vi "SV RMS Average Spectra (Real).vi"(0 "real spectra":cluster{"f0":dbl, "df":dbl, "magnitude":dbl[]}[](array[cluster]) {"magnitude" format="%.2p"; "df" format="%.2p"; "f0" format="%.2p"}, 4 "spectrum info":T1={"channel name"="", "description"="", "x-axis units"=0, "spectral info"={"spectrum type"=enum."Power [Magnitude^2]", "linear/dB"=enum."linear", "window"=0, "window size"=0, "FFT size"=0}, "engineering units"=1, "custom label"="", "dB reference [EU]"=0.0, "peak units"=enum."rms", "weighting filter"=0, "spectral density?"=FALSE, "unit label"="", "spectrum skewed?"=FALSE, "complimentary spectrum units"=enum."none"} {"x-axis units" items=["Time (s)"=0, "Frequency-CB (Hz)"=1, "Frequency-CPB (Hz)"=1248, "Frequency-Arbitrary (Hz)"=2357, "Quefrency (s)"=2, "Revolutions (rev)"=3, "Order"=4, "Speed (RPM)"=11, "Speed (rad/s)"=21, "Index"=65535]; "weighting filter" items=["Linear", "A-weighting", "B-weighting", "C-weighting", "ITU-R 468-4", "Dolby", "CCITT", "C-message", "Wb", "Wc", "Wd", "We", "Wf", "Wh", "Wj", "Wk", "Wm", "AES17 20 kHz lowpass", "AES17 40 kHz lowpass", "AES17 20 kHz highpass", "AES17 40 kHz highpass"]; "dB reference [EU]" format="%.2f"; "engineering units" items=["custom..."=0, "V"=1, "A"=21, "C"=30, "pC"=31, "s"=32, "-"=29, "Pa"=2, "N"=20, "g"=3, "m/s^2"=4, "m/s"=5, "m"=6, "mm/s"=12, "mm"=13, "micron/s"=14, "micron"=15, "in/s^2"=7, "in/s"=8, "in"=9, "mil/s"=10, "mil"=11, "rad/s^2"=16, "rad/s"=17, "rad"=18, "deg/s^2"=26, "deg/s"=27, "deg"=28, "RPM"=22, "cycle/s^2"=23, "Hz"=24, "cycle"=25, "strain"=19]; "spectral info"."window" items=["None "=0, "Hanning"=1, "Hamming"=2, "Blackman-Harris"=3, "Exact Blackman"=4, "Blackman"=5, "Flat Top"=6, "4 Term B-Harris "=7, "7 Term B-Harris"=8, "Low Sidelobe"=9, "Force - Exponential"=10, "Gaussian"=62]}, 5 "error in (no error)":errorcluster) -> (13 "averages completed":dbl, 14 "rms average spectrum":cluster{"f0":dbl, "df":dbl, "magnitude":dbl[]} {"magnitude" format="%.2p"; "df" format="%.2p"; "f0" format="%.2p"}, 15 "unit label":string, 18 "spectrum info":T1={"channel name"="", "description"="", "x-axis units"=0, "spectral info"={"spectrum type"=enum."Power [Magnitude^2]", "linear/dB"=enum."linear", "window"=0, "window size"=0, "FFT size"=0}, "engineering units"=1, "custom label"="", "dB reference [EU]"=0.0, "peak units"=enum."rms", "weighting filter"=0, "spectral density?"=FALSE, "unit label"="", "spectrum skewed?"=FALSE, "complimentary spectrum units"=enum."none"} {"x-axis units" items=["Time (s)"=0, "Frequency-CB (Hz)"=1, "Frequency-CPB (Hz)"=1248, "Frequency-Arbitrary (Hz)"=2357, "Quefrency (s)"=2, "Revolutions (rev)"=3, "Order"=4, "Speed (RPM)"=11, "Speed (rad/s)"=21, "Index"=65535]; "weighting filter" items=["Linear", "A-weighting", "B-weighting", "C-weighting", "ITU-R 468-4", "Dolby", "CCITT", "C-message", "Wb", "Wc", "Wd", "We", "Wf", "Wh", "Wj", "Wk", "Wm", "AES17 20 kHz lowpass", "AES17 40 kHz lowpass", "AES17 20 kHz highpass", "AES17 40 kHz highpass"]; "dB reference [EU]" format="%.2f"; "engineering units" items=["custom..."=0, "V"=1, "A"=21, "C"=30, "pC"=31, "s"=32, "-"=29, "Pa"=2, "N"=20, "g"=3, "m/s^2"=4, "m/s"=5, "m"=6, "mm/s"=12, "mm"=13, "micron/s"=14, "micron"=15, "in/s^2"=7, "in/s"=8, "in"=9, "mil/s"=10, "mil"=11, "rad/s^2"=16, "rad/s"=17, "rad"=18, "deg/s^2"=26, "deg/s"=27, "deg"=28, "RPM"=22, "cycle/s^2"=23, "Hz"=24, "cycle"=25, "strain"=19]; "spectral info"."window" items=["None "=0, "Hanning"=1, "Hamming"=2, "Blackman-Harris"=3, "Exact Blackman"=4, "Blackman"=5, "Flat Top"=6, "4 Term B-Harris "=7, "7 Term B-Harris"=8, "Low Sidelobe"=9, "Force - Exponential"=10, "Gaussian"=62]}, 19 "error out":errorcluster)   [LabVIEW 2017]
doc: "Computes the linear RMS-averaged power spectrum of <B>scaled signal [EU]</B> in a linear scale. Use the power spectrum to quantify signal components as a function of frequency. Use this VI on embedded targets that have limited computational resources. Wire data to the <B>scaled signal [EU]</B> input to determine the polymorphic instance to use or manually select the instance."
uses:
  <vilib>/addons/_NISVFA/_Shared subVIs/Controls/svc_Spectrum Info.ctl
  <vilib>/addons/_NISVFA/_Shared subVIs/Controls/svc_X-Axis Units.ctl
  <vilib>/addons/_NISVFA/_Shared subVIs/Controls/svc_Spectrum Type.ctl
  <vilib>/addons/_NISVFA/_Shared subVIs/Controls/svc_Engineering Units Text Ring.ctl
  <vilib>/addons/_NISVFA/_Shared subVIs/Controls/svc_Weighting Filter Text Ring.ctl
  <vilib>/addons/_NISVFA/_Shared subVIs/Controls/svc_Complimentary Spectrum Units.ctl
  <vilib>/addons/_NISVFA/_Spectrum Processing/SVFA Unit Conversion (1 Ch).vi
  <vilib>/addons/_NISVFA/_Shared subVIs/Common/svc_Spectrum Units.vi
  <vilib>/addons/_NISVFA/_Spectrum Processing/subVIs/svfa_Conversion Utility (spectrum info).vi
  <vilib>/addons/_NISVFA/_Spectrum Processing/subVIs/svfa_Peak to RMS to Peak2Peak.vi
  <vilib>/addons/_NISVFA/_Spectrum Processing/subVIs/svfa_Mag to Mag2.vi
  <vilib>/addons/_NISVFA/_Spectrum Processing/subVIs/svfa_Linear to dB.vi
  <vilib>/addons/_NISVFA/_Spectrum Processing/subVIs/svfa_dBrefA to dBrefB.vi
  <vilib>/addons/_NISVFA/_Spectrum Processing/subVIs/svfa_Spectrum to Spectral Density.vi
  <vilib>/addons/_NISVFA/_Shared subVIs/Common/svc_Get Weighting Enum and Labels.vi
  <vilib>/addons/_NISVFA/_Shared subVIs/Common/svc_Unit Label Lexical Class.vi
  <vilib>/addons/_NISVFA/_Shared subVIs/Common/svc_Engineering Units to Unit Label.vi
  <vilib>/addons/_NISVFA/_Shared subVIs/Common/svc_Format Value (DBL).vi
  <vilib>/addons/_NISVFA/_Shared subVIs/Common/svc_Window Parameters.vi
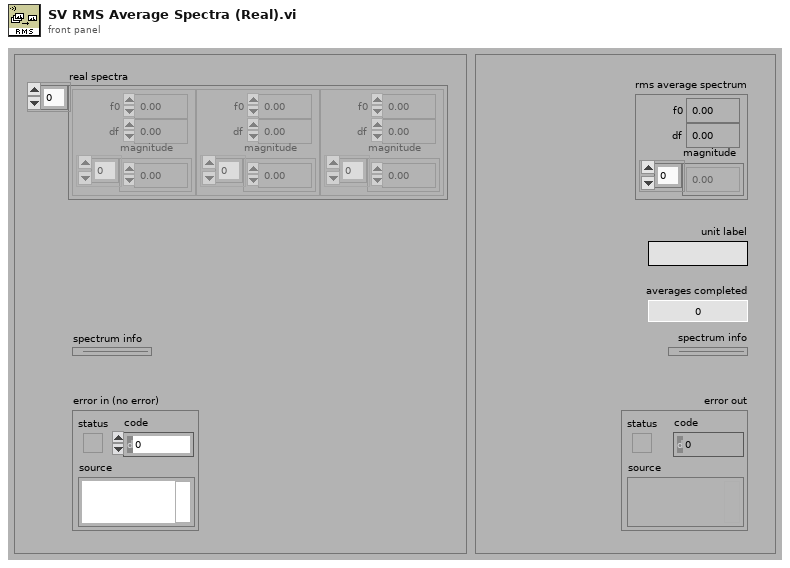
[diagram p1: front panel]
types:
  T1 = typedef "svc_Spectrum Info.ctl" = cluster{"channel name":string, "description":string, "x-axis units":T2, "spectral info":cluster{"spectrum type":T3, "linear/dB":enum16{"linear", "dB"}, "window":u16, "window size":i32, "FFT size":i32}, "engineering units":T4, "custom label":string, "dB reference [EU]":dbl, "peak units":enum16{"rms", "peak", "peak-peak"}, "weighting filter":T5, "spectral density?":bool, "unit label":string, "spectrum skewed?":bool, "complimentary spectrum units":T6}
  T2 = typedef "svc_X-Axis Units.ctl" = u16
  T3 = typedef "svc_Spectrum Type.ctl" = enum16{"FFT Spectrum [complex]", "Amplitude [Magnitude]", "Power [Magnitude^2]", "Cross Spectrum [complex]", "Frequency Response [Complex]"}
  T4 = typedef "svc_Engineering Units Text Ring.ctl" = u16
  T5 = typedef "svc_Weighting Filter Text Ring.ctl" = u16
  T6 = typedef "svc_Complimentary Spectrum Units.ctl" = enum16{"none", "radians", "degrees", "cycles", "imaginary"}
  T7 = cluster{"linear/dB":enum16{"no change", "linear", "dB"}, "dB reference (0: no change)":dbl, "power/magnitude":enum16{"no change", "power", "magnitude"}, "view":enum16{"no change", "rms", "peak", "peak-peak"}}
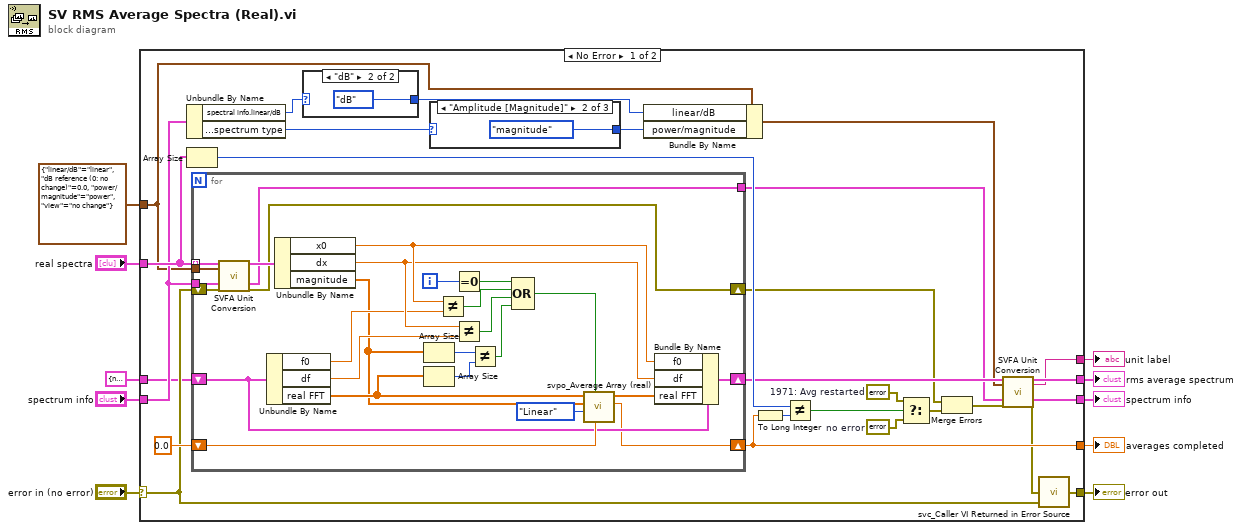
[diagram p0: block diagram]
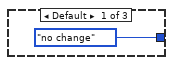
[diagram p2: hidden frame]
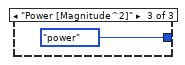
[diagram p3: hidden frame]
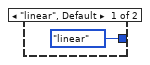
[diagram p4: hidden frame]
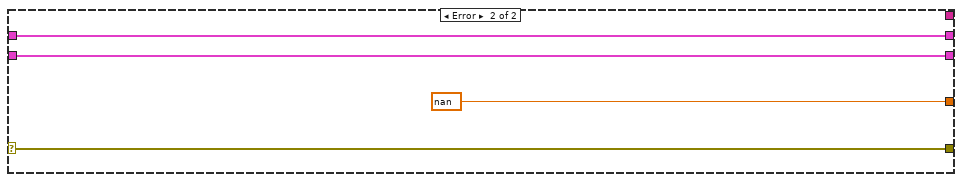
[diagram p5: hidden frame]
diagram:
  n1 = case shown="No Error" "error in (no error)" {
    selector: "error in (no error)" -> [w28 w72]
    tunnel: [w23 w70] -> w10
    tunnel: "real spectra" -> [w29 _]
    tunnel: [w36 nan ("Numeric")] -> w8
    tunnel: "spectrum info" -> [w27 w71]
    tunnel: [w30 w72] -> w5
    tunnel: [w22 w71] -> w4
    tunnel: T7 {"linear/dB"=enum."linear", "dB reference (0: no change)"=0.0, "power/magnitude"=enum."power", "view"=enum."no change"} ("desired scaling") -> [w13 _]
    tunnel: [w14 _] -> w2
    tunnel: cluster{"f0":dbl, "df":dbl, "real FFT":dbl[]} {"f0"=nan, "df"=nan, "real FFT"=[]} ("previous avg real spectrum") -> [w11 w70]
    frame No Error {
      w32 = errorcluster {"status"=FALSE, "code"=0, "source"=""}  # no error
      w33 = errorcluster {"status"=FALSE, "code"=1971, "source"="<append>\n\nAveraging restarted due to change in f0, df, or spectrum size within real spectra input."}  # 1971: Avg restarted
      n2 = Unbundle By Name(w27) -> ("spectral info.linear/dB"=w26:enum16{"linear", "dB"}, "spectral info.spectrum type"=w25:T3)
      n3 = Array Size(array=w29) -> (size(s)=w35:i32)
      n4 = for {
        tunnel: w29 -> [w52] mode=indexing
        shift-right: [w55] -> w36
        shift-left: 0.0 ("Numeric") -> [w63]
        shift-right: [w56] -> w24
        shift-left: w11 -> [w60]
        tunnel: w27 -> [w50]
        tunnel: w13 -> [w49]
        shift-right: [w47] -> w21
        shift-left: w28 -> [w48]
        tunnel: [w46] -> w18
        i -> [w61]
        n5 = call-poly <vilib>:"SVFA Unit Conversion.vi"("spectrum"=w52, "desired scaling"=w49, "spectrum info in"=w50, "error in (no error)"=w48) -> ("converted spectrum"=w51:cluster{"x0":dbl, "dx":dbl, "magnitude":dbl[]}, "spectrum info out"=w46:T1, "error out"=w47:errorcluster)  [unwired: 12 in, 1 out]
        n6 = Unbundle By Name(w60) -> ("f0"=w54:dbl, "df"=w53:dbl, "real FFT"=w44:dbl[])
        n7 = Unbundle By Name(w51) -> ("x0"=w58:dbl, "dx"=w57:dbl, "magnitude"=w43:dbl[])
        n8 = Array Size(array=w43) -> (size(s)=w69:i32)
        n9 = Array Size(array=w44) -> (size(s)=w68:i32)
        n10 = Not Equal?(x=w58, y=w54) -> (x != y?=w67:bool)
        n11 = Equal To 0?(x=w61) -> (x = 0?=w62:bool)
        n12 = Not Equal?(x=w57, y=w53) -> (x != y?=w65:bool)
        n13 = Not Equal?(x=w69, y=w68) -> (x != y?=w66:bool)
        n14 = Compound Arithmetic op=OR(w62, w67, w65, w66) -> (w45:bool)
        n15 = call <vilib>:"svpo_Average Array (real).vi"("averages completed in"=w63, "restart averaging"=w45, "weighting mode"=enum16{"Linear", "Exponential"}."Linear", "array"=w43, "previous average array"=w44) -> ("averages completed out"=w55:dbl, "average array"=w59:dbl[])  [unwired: 5 in]
        n16 = Bundle By Name(cluster=w60, "f0"=w58, "df"=w57, "real FFT"=w59) -> (w56:cluster{"f0":dbl, "df":dbl, "real FFT":dbl[]})
      }
      n17 = case shown="\"dB\"" w26 {
        tunnel: [enum16{"no change", "linear", "dB"}."linear" ("linear/dB") enum16{"no change", "linear", "dB"}."dB" ("linear/dB")] -> w16
        frame "linear", Default {
        }
        frame "dB" {
        }
      }
      n18 = case shown="\"Amplitude [Magnitude]\"" w25 {
        tunnel: [enum16{"no change", "power", "magnitude"}."no change" ("power/magnitude") enum16{"no change", "power", "magnitude"}."magnitude" ("power/magnitude") enum16{"no change", "power", "magnitude"}."power" ("power/magnitude")] -> w17
        frame Default {
        }
        frame "Amplitude [Magnitude]" {
        }
        frame "Power [Magnitude^2]" {
        }
      }
      n19 = Bundle By Name(cluster=w13, "linear/dB"=w16, "power/magnitude"=w17) -> (w15:T7)
      n20 = To Long Integer(number=w36) -> (32bit integer=w34:i32)
      n21 = Not Equal?(x=w35, y=w34) -> (x != y?=w31:bool)
      n22 = Select(t=w33, s=w31, f=w32) -> (s? t:f=w20:errorcluster)
      n23 = Merge Errors(w21, w20) -> (w19:errorcluster)
      n24 = call-poly <vilib>:"SVFA Unit Conversion.vi"("spectrum"=w24, "desired scaling"=w15, "spectrum info in"=w18, "error in (no error)"=w19) -> ("converted spectrum"=w23:cluster{"x0":dbl, "dx":dbl, "magnitude":dbl[]}, "unit label"=w14:string, "spectrum info out"=w22:T1, "error out"=w12:errorcluster)  [unwired: 12 in]
      n25 = call <vilib>:"svc_Caller VI Returned in Error Source.vi"("warning input to caller"=w28, "error in (no error)"=w12) -> ("error out"=w30:errorcluster)  [unwired: 3 in]
    }
    frame Error {
    }
  }
  "rms average spectrum" <- w10
  "averages completed" <- w8
  "error out" <- w5
  "spectrum info" <- w4
  "unit label" <- w2
